vi "set_temperature_value.vi"   [LabVIEW 2019]
uses:
  global_temperature_cluster.ctl
  Instrument_Setup.vi
  Global/Global Variables/Data_Display_global.vi
  Global_temperature_variables.vi
types:
  T1 = typedef "global_temperature_cluster.ctl" = cluster{"370-T1":dbl, "370-T2":dbl, "370-T3":dbl, "370-T4":dbl, "370-T5":dbl, "372-T1":dbl, "372-T2":dbl, "372-T3":dbl, "372-T4":dbl, "372-T5":dbl, "372-T6":dbl, "350-T1":dbl, "350-T2":dbl, "350-T3":dbl, "350-T4":dbl, "VTI CH1":dbl, "VTI CH2":dbl, "VTI CH3":dbl, "AVS Control Channel (K)":dbl}
  T2 = typedef "PicowattAVS47-Cluster.ctl" = cluster{"Control Channel (K)":dbl, "AVS CH 5 (Res)":dbl, "AVS CH 6 (Res) ":dbl, "AVS CH 7 (Res) ":dbl, "Control Res.":dbl, "Auto Excitation":bool, "Auto activatet":bool, "AVS Excitation":i16}
  T3 = typedef "ITC503Monitor-Cluster.ctl" = cluster{"Temperatur (K)":dbl, "Setpoint (K)":dbl, "Rate (K/min)":dbl, "Heater (%)":dbl, "NV (%)":dbl, "Heater Manual":bool, "NV Manual":bool, "Go to Set":bool, "Heater SP":dbl, "Valid?":bool, "Set Heater SP":bool, "Set NV SP":bool, "Heater (%) Display":dbl, "NV (%) Display":dbl, "NV Setpoint":dbl, "Change Heater Status":bool, "Change NV Status":bool, "Sample 3":dbl, "Sample 2":dbl, "Sweep-State":bool, "Set Auto PID":bool, "Auto PID":bool, "Stopp":bool, "Setpoint-Sweep":dbl, "Sample 1":dbl, "Control Channel":bool, "Channel 1":bool, "Channel 2":bool, "Channel 3":bool}
  T4 = typedef "LS370_only_readout_cluster.ctl" = cluster{"LS370 T1":dbl, "LS370 T2":dbl, "LS370 T3":dbl, "LS370 T4":dbl, "LS370 T5":dbl, "LS370 R1":dbl, "LS370 R2":dbl, "LS370 R3":dbl, "LS370 R4":dbl, "LS370 R5":dbl, "LS370 T6":dbl, "LS370 T7":dbl, "LS370 T8":dbl, "LS370 T9":dbl, "LS370 R6":dbl, "LS370 R7":dbl, "LS370 R8":dbl, "LS370 R9":dbl, "LS370 TC-T":dbl, "LS370 TC-R":dbl, "Update Lakeshores":bool}
  T5 = typedef "LS372_read_only-Cluster.ctl" = cluster{"LS372-T1":dbl, "LS372 -T2":dbl, "LS372-T4":dbl, "LS372-T5":dbl, "LS372-T6":dbl, "LS372-R1 ":dbl, "LS372-R2":dbl, "LS372-R3 ":dbl, "LS372-R4 \n\n\n\n":dbl, "LS372-R5":dbl, "LS372-R6 ":dbl, "LS372-T3":dbl, "Update Lakeshores":bool}
  T6 = typedef "LS350-cluster.ctl" = cluster{"Setpoint":dbl, "Heater Output":dbl, "Setpoint control":dbl, "Enable Setpoint":bool, "LS350 T1":dbl, "LS350 T2":dbl, "LS350 T3":dbl, "LS350 T4":dbl, "LS350 R1":dbl, "LS350 R2":dbl, "LS350 R3":dbl, "LS350 R4":dbl}
  T7 = typedef "VTI-cluster.ctl" = cluster{"Temperatur (K)":dbl, "Setpoint (K)":dbl, "Rate (K/min)":dbl, "Heater (%)":dbl, "NV (%)":dbl, "Heater Manual":bool, "NV Manual":bool, "Go to Set":bool, "Pressure":dbl, "Heater SP":dbl, "Valid?":bool, "Set Heater SP":bool, "Set NV SP":bool, "Heater (%) Display":dbl, "NV (%) Display":dbl, "NV Setpoint":dbl, "Change Heater Status":bool, "Change NV Status":bool, "Sample 3":dbl, "Sample 2":dbl, "Sweep-State":bool, "Set Auto PID":bool, "Auto PID":bool, "Stopp":bool, "Setpoint-Sweep":dbl}
  T8 = typedef "LS370_Status.ctl" = cluster{"Setpoint":dbl, "MC Heater Output":dbl, "Still Heater Output":dbl, "Sorb  Heater Output":dbl, "LS370 T1":dbl, "LS370 T2":dbl, "LS370 T3":dbl, "LS370 T4":dbl, "LS370 T5":dbl, "LS370 R1":dbl, "LS370 R2":dbl, "LS370 R3":dbl, "LS370 R4":dbl, "LS370 R5":dbl, "LS370 T6":dbl, "LS370 T7":dbl, "LS370 T8":dbl, "LS370 T9":dbl, "LS370 R6":dbl, "LS370 R7":dbl, "LS370 R8":dbl, "LS370 R9":dbl, "LS370 TC-T":dbl, "LS370 TC-R":dbl}
  T9 = typedef "LS372-Cluster.ctl" = cluster{"Activate Tsweep":bool, "Setpoint - Manual":dbl, "Rate (K/min)":dbl, "Update Lakeshores":bool, "Still Heater":bool, "Still Power (mW)":dbl, "Manual Heater":bool, "Manual Heater  (mW) ":dbl, "Heater Range":dbl, "P (Gain)":dbl, "I (Reset)":dbl, "D (Rate)":dbl, "Heater Power (mW)":dbl, "MC Thermometer":u16, "MC Temperature":dbl, "LS372-T1":dbl, "LS372 -T2":dbl, "LS372-R1 ":dbl, "LS372-R2":dbl, "LS372-T3":dbl, "LS372-T4":dbl, "LS372-R3 ":dbl, "LS372-R4 \n\n\n\n":dbl, "LS372-T5":dbl, "LS372-T6":dbl, "LS372-R5":dbl, "LS372-R6 ":dbl, "Still Power ist":dbl, "Set Temperatur Sweep main":bool, "Setpoint ist":dbl, "Disable Heater":bool}
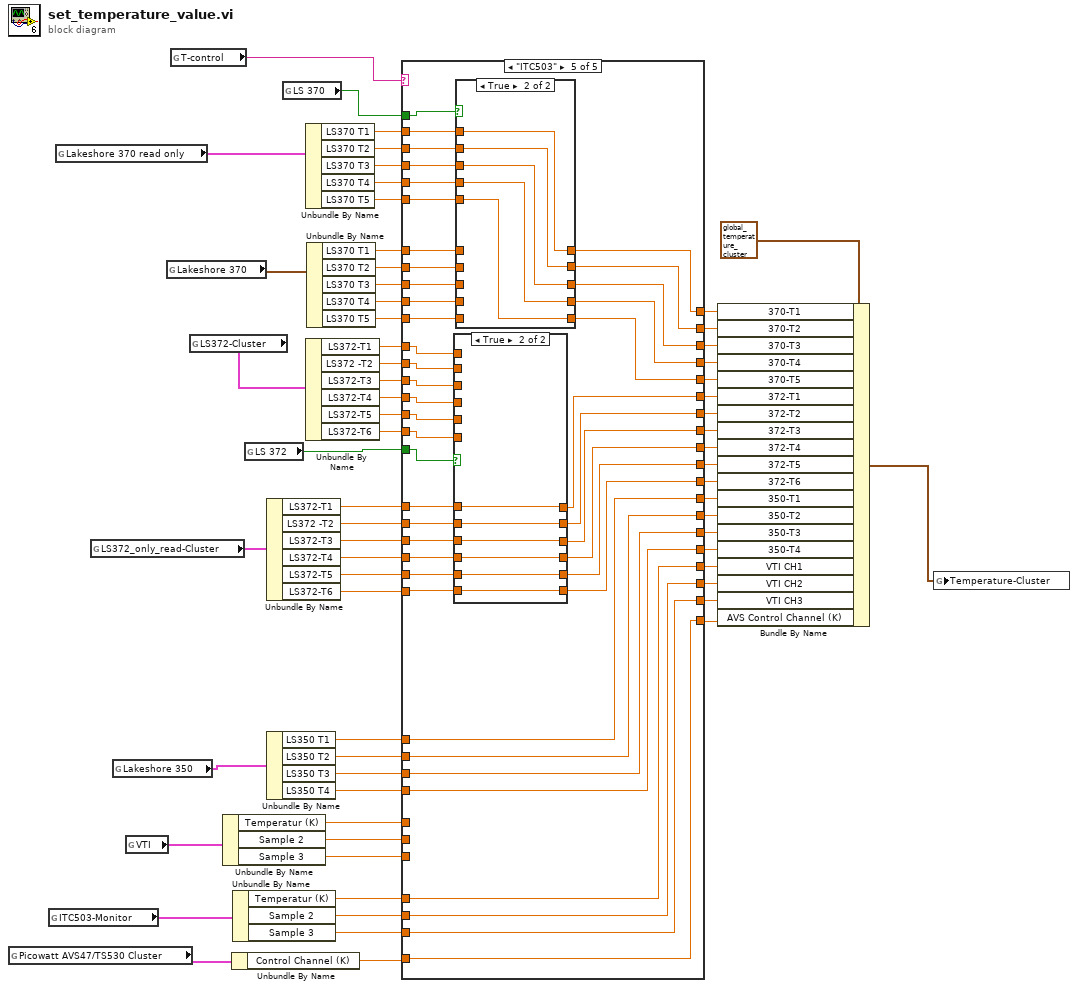
[diagram p0: block diagram]
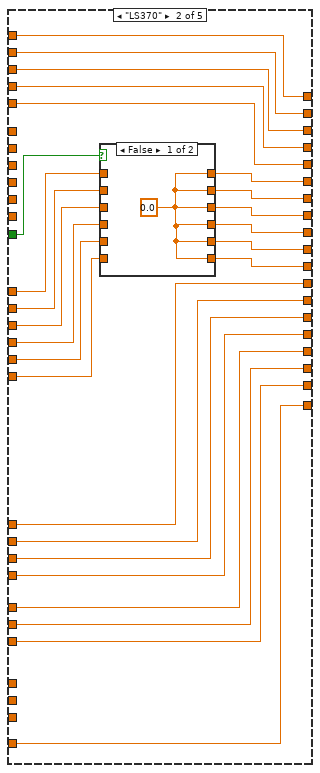
[diagram p5: hidden frame]
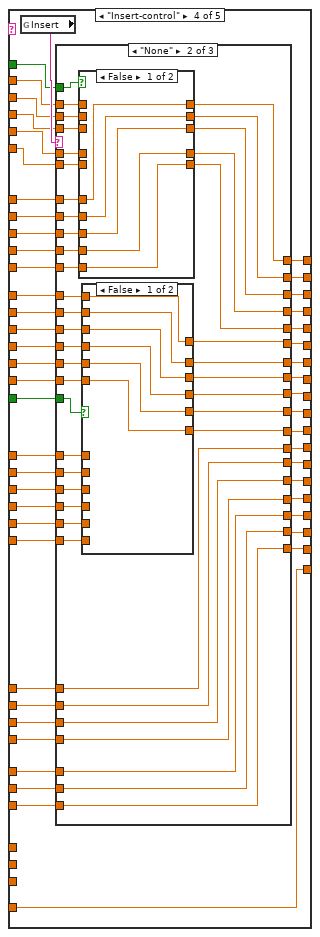
[diagram p9: hidden frame]
diagram:
  n1 = global read "Data_Display_global.vi" "Picowatt AVS47/TS530 Cluster"() -> (w56:T2)
  n2 = global read "Data_Display_global.vi" "ITC503-Monitor"() -> (w32:T3)
  n3 = global read "Data_Display_global.vi" "Lakeshore 370 read only"() -> (w7:T4)
  n4 = global read "Data_Display_global.vi" "LS372_only_read-Cluster"() -> (w57:T5)
  n5 = global read "Data_Display_global.vi" "Lakeshore 350"() -> (w58:T6)
  n6 = global read "Data_Display_global.vi" "VTI"() -> (w59:T7)
  n7 = global read "Data_Display_global.vi" "Lakeshore 370"() -> (w60:T8)
  n8 = global read "Instrument_Setup.vi" "T-control"() -> (w63:string)
  n9 = global read "Data_Display_global.vi" "LS372-Cluster"() -> (w61:T9)
  n10 = Unbundle By Name(w59) -> ("Temperatur (K)"=w33:dbl, "Sample 2"=w34:dbl, "Sample 3"=w35:dbl)
  n11 = Unbundle By Name(w56) -> ("Control Channel (K)"=w36:dbl)
  n12 = Unbundle By Name(w32) -> ("Temperatur (K)"=w31:dbl, "Sample 2"=w30:dbl, "Sample 3"=w29:dbl)
  n13 = global read "Instrument_Setup.vi" "LS 372"() -> (w62:bool)
  n14 = Unbundle By Name(w57) -> ("LS372-T1"=w17:dbl, "LS372 -T2"=w16:dbl, "LS372-T3"=w15:dbl, "LS372-T4"=w14:dbl, "LS372-T5"=w13:dbl, "LS372-T6"=w12:dbl)
  n15 = Unbundle By Name(w58) -> ("LS350 T1"=w11:dbl, "LS350 T2"=w10:dbl, "LS350 T3"=w9:dbl, "LS350 T4"=w8:dbl)
  n16 = global read "Instrument_Setup.vi" "LS 370"() -> (w1:bool)
  n17 = Unbundle By Name(w7) -> ("LS370 T1"=w6:dbl, "LS370 T2"=w5:dbl, "LS370 T3"=w4:dbl, "LS370 T4"=w3:dbl, "LS370 T5"=w2:dbl)
  n18 = Unbundle By Name(w61) -> ("LS372-T1"=w23:dbl, "LS372 -T2"=w22:dbl, "LS372-T3"=w21:dbl, "LS372-T4"=w20:dbl, "LS372-T5"=w19:dbl, "LS372-T6"=w18:dbl)
  n19 = Unbundle By Name(w60) -> ("LS370 T1"=w28:dbl, "LS370 T2"=w27:dbl, "LS370 T3"=w26:dbl, "LS370 T4"=w25:dbl, "LS370 T5"=w24:dbl)
  n20 = case shown="\"ITC503\"" w63 {
    tunnel: w62 -> [w92 w156 _ w248 w452]
    tunnel: [w97 w151 w187 w235 w457] -> w55
    tunnel: [w96 w150 w186 w234 w456] -> w54
    tunnel: [w95 w149 w185 w233 w455] -> w53
    tunnel: [w94 w148 w184 w232 w454] -> w52
    tunnel: [w93 w147 w183 w231 w453] -> w51
    tunnel: [w79 w146 w177 w230 w439] -> w50
    tunnel: [w78 w145 w176 w229 w438] -> w49
    tunnel: [w77 w144 w175 w228 w437] -> w48
    tunnel: [w76 w143 w174 w227 w436] -> w47
    tunnel: [w75 w142 w173 w226 w435] -> w46
    tunnel: [w74 w141 w172 w225 w434] -> w45
    tunnel: [w73 w140 w171 w217 w433] -> w44
    tunnel: [w72 w137 w170 w216 w432] -> w43
    tunnel: [w71 w139 w169 w215 w431] -> w42
    tunnel: [w70 w138 w168 w214 w430] -> w41
    tunnel: [w69 w152 w167 w213 w429] -> w40
    tunnel: [w68 w153 w166 w212 w428] -> w39
    tunnel: [w67 w154 w165 w211 w427] -> w38
    tunnel: [w66 w155 w164 w210 w426] -> w37
    tunnel: w36 -> [w66 w155 w164 w210 w426]
    tunnel: w35 -> [w67 w154 w165 w218 _]
    tunnel: w34 -> [w68 w153 w166 w219 _]
    tunnel: w33 -> [w69 w152 w167 w220 _]
    tunnel: w31 -> [_ _ _ _ w429]
    tunnel: w30 -> [_ _ _ _ w428]
    tunnel: w29 -> [_ _ _ _ w427]
    tunnel: w28 -> [w102 w151 w182 w253 w462]
    tunnel: w27 -> [w101 w150 w181 w252 w461]
    tunnel: w26 -> [w100 w149 w180 w251 w460]
    tunnel: w25 -> [w99 w148 w179 w250 w459]
    tunnel: w24 -> [w98 w147 w178 w249 w458]
    tunnel: w23 -> [w91 _ w177 w247 w451]
    tunnel: w22 -> [w90 _ w176 w246 w450]
    tunnel: w21 -> [w89 _ w175 w245 w449]
    tunnel: w20 -> [w88 _ w174 w244 w448]
    tunnel: w19 -> [w87 _ w173 w243 w447]
    tunnel: w18 -> [w86 _ w172 w242 w446]
    tunnel: w17 -> [w85 w131 _ w241 w445]
    tunnel: w16 -> [w84 w132 _ w240 w444]
    tunnel: w15 -> [w83 w133 _ w239 w443]
    tunnel: w14 -> [w82 w134 _ w238 w442]
    tunnel: w13 -> [w81 w135 _ w237 w441]
    tunnel: w12 -> [w80 w136 _ w236 w440]
    tunnel: w11 -> [w73 w140 w171 w224 w433]
    tunnel: w10 -> [w72 w137 w170 w223 w432]
    tunnel: w9 -> [w71 w139 w169 w222 w431]
    tunnel: w8 -> [w70 w138 w168 w221 w430]
    tunnel: w6 -> [w107 _ w192 w208 w467]
    tunnel: w5 -> [w106 _ w191 w207 w466]
    tunnel: w4 -> [w105 _ w190 w206 w465]
    tunnel: w3 -> [w104 _ w189 w205 w464]
    tunnel: w2 -> [w103 _ w188 w204 w463]
    tunnel: w1 -> [w108 _ w193 w209 w468]
    frame "None", Default {
      n21 = case shown="False" w92 {
        tunnel: w91 -> [w114 _]
        tunnel: w90 -> [w113 _]
        tunnel: w89 -> [w112 _]
        tunnel: w88 -> [w111 _]
        tunnel: w87 -> [w110 _]
        tunnel: w86 -> [w109 _]
        tunnel: w85 -> [_ w120]
        tunnel: w84 -> [_ w119]
        tunnel: w83 -> [_ w118]
        tunnel: w82 -> [_ w117]
        tunnel: w81 -> [_ w116]
        tunnel: w80 -> [_ w115]
        tunnel: [w114 w120] -> w79
        tunnel: [w113 w119] -> w78
        tunnel: [w112 w118] -> w77
        tunnel: [w111 w117] -> w76
        tunnel: [w110 w116] -> w75
        tunnel: [w109 w115] -> w74
        frame False {
        }
        frame True {
        }
      }
      n22 = case shown="False" w108 {
        tunnel: w107 -> [_ w130]
        tunnel: w106 -> [_ w129]
        tunnel: w105 -> [_ w128]
        tunnel: w104 -> [_ w127]
        tunnel: w103 -> [_ w126]
        tunnel: [w125 w130] -> w97
        tunnel: [w124 w129] -> w96
        tunnel: [w123 w128] -> w95
        tunnel: [w122 w127] -> w94
        tunnel: [w121 w126] -> w93
        tunnel: w102 -> [w125 _]
        tunnel: w101 -> [w124 _]
        tunnel: w100 -> [w123 _]
        tunnel: w99 -> [w122 _]
        tunnel: w98 -> [w121 _]
        frame False {
        }
        frame True {
        }
      }
    }
    frame "LS370" {
      n23 = case shown="False" w156 {
        tunnel: w131 -> [_ w163]
        tunnel: w132 -> [_ w162]
        tunnel: w133 -> [_ w161]
        tunnel: w134 -> [_ w160]
        tunnel: w135 -> [_ w159]
        tunnel: w136 -> [_ w158]
        tunnel: [w157 w163] -> w146
        tunnel: [w157 w162] -> w145
        tunnel: [w157 w161] -> w144
        tunnel: [w157 w160] -> w143
        tunnel: [w157 w159] -> w142
        tunnel: [w157 w158] -> w141
        frame False {
          w157 = 0.0
        }
        frame True {
        }
      }
    }
    frame "LS372" {
      n24 = case shown="False" w193 {
        tunnel: w192 -> [_ w203]
        tunnel: w191 -> [_ w202]
        tunnel: w190 -> [_ w201]
        tunnel: w189 -> [_ w200]
        tunnel: w188 -> [_ w199]
        tunnel: [w198 w203] -> w187
        tunnel: [w197 w202] -> w186
        tunnel: [w196 w201] -> w185
        tunnel: [w195 w200] -> w184
        tunnel: [w194 w199] -> w183
        tunnel: w182 -> [w198 _]
        tunnel: w181 -> [w197 _]
        tunnel: w180 -> [w196 _]
        tunnel: w179 -> [w195 _]
        tunnel: w178 -> [w194 _]
        frame False {
        }
        frame True {
        }
      }
    }
    frame "Insert-control" {
      n25 = global read "Instrument_Setup.vi" "Insert"() -> (w254:string)
      n26 = case shown="\"None\"" w254 {
        tunnel: w253 -> [w290 w354 w400]
        tunnel: w252 -> [w289 w353 w399]
        tunnel: w251 -> [w288 w352 w398]
        tunnel: w250 -> [w287 w351 w397]
        tunnel: w249 -> [w286 w350 w396]
        tunnel: w248 -> [w274 w344 w413]
        tunnel: w247 -> [w280 w343 w412]
        tunnel: w246 -> [w279 w342 w411]
        tunnel: w245 -> [w278 w341 w410]
        tunnel: w244 -> [w277 w340 w409]
        tunnel: w243 -> [w276 w339 w408]
        tunnel: w242 -> [w275 w338 w407]
        tunnel: w241 -> [w273 w337 w406]
        tunnel: w240 -> [w272 w336 w405]
        tunnel: w239 -> [w271 w335 w404]
        tunnel: w238 -> [w270 w334 w403]
        tunnel: w237 -> [w269 w333 w402]
        tunnel: w236 -> [w268 w332 w401]
        tunnel: [w285 w349 w400] -> w235
        tunnel: [w284 w348 w399] -> w234
        tunnel: [w283 w347 w398] -> w233
        tunnel: [w282 w346 w397] -> w232
        tunnel: [w281 w345 w396] -> w231
        tunnel: [w267 w331 w395] -> w230
        tunnel: [w266 w330 w394] -> w229
        tunnel: [w265 w329 w393] -> w228
        tunnel: [w264 w328 w392] -> w227
        tunnel: [w263 w327 w391] -> w226
        tunnel: [w262 w326 w390] -> w225
        tunnel: w224 -> [w261 w325 w389]
        tunnel: w223 -> [w260 w324 w388]
        tunnel: w222 -> [w259 w323 w387]
        tunnel: w221 -> [w258 w322 w386]
        tunnel: [w261 w325 w389] -> w217
        tunnel: [w260 w324 w388] -> w216
        tunnel: [w259 w323 w387] -> w215
        tunnel: [w258 w322 w386] -> w214
        tunnel: w220 -> [w257 w321 w385]
        tunnel: w219 -> [w256 w320 w384]
        tunnel: w218 -> [w255 w319 w383]
        tunnel: [w257 w321 w385] -> w213
        tunnel: [w256 w320 w384] -> w212
        tunnel: [w255 w319 w383] -> w211
        tunnel: w209 -> [w296 w360 _]
        tunnel: w208 -> [w295 w359 _]
        tunnel: w207 -> [w294 w358 _]
        tunnel: w206 -> [w293 w357 _]
        tunnel: w205 -> [w292 w356 _]
        tunnel: w204 -> [w291 w355 _]
        frame "VTI", Default {
          n27 = case shown="False" w296 {
            tunnel: w295 -> [_ w318]
            tunnel: w294 -> [_ w317]
            tunnel: w293 -> [_ w316]
            tunnel: w292 -> [_ w315]
            tunnel: w291 -> [_ w314]
            tunnel: w290 -> [w313 _]
            tunnel: w289 -> [w312 _]
            tunnel: w288 -> [w311 _]
            tunnel: w287 -> [w310 _]
            tunnel: w286 -> [w309 _]
            tunnel: [w313 w318] -> w285
            tunnel: [w312 w317] -> w284
            tunnel: [w311 w316] -> w283
            tunnel: [w310 w315] -> w282
            tunnel: [w309 w314] -> w281
            frame False {
            }
            frame True {
            }
          }
          n28 = case shown="True" w274 {
            tunnel: w280 -> [w302 _]
            tunnel: w279 -> [w301 _]
            tunnel: w278 -> [w300 _]
            tunnel: w277 -> [w299 _]
            tunnel: w276 -> [w298 _]
            tunnel: w275 -> [w297 _]
            tunnel: w273 -> [_ w308]
            tunnel: w272 -> [_ w307]
            tunnel: w271 -> [_ w306]
            tunnel: w270 -> [_ w305]
            tunnel: w269 -> [_ w304]
            tunnel: w268 -> [_ w303]
            tunnel: [w302 w308] -> w267
            tunnel: [w301 w307] -> w266
            tunnel: [w300 w306] -> w265
            tunnel: [w299 w305] -> w264
            tunnel: [w298 w304] -> w263
            tunnel: [w297 w303] -> w262
            frame False {
            }
            frame True {
            }
          }
        }
        frame "None" {
          n29 = case shown="False" w360 {
            tunnel: w359 -> [_ w382]
            tunnel: w358 -> [_ w381]
            tunnel: w357 -> [_ w380]
            tunnel: w356 -> [_ w379]
            tunnel: w355 -> [_ w378]
            tunnel: w354 -> [w377 _]
            tunnel: w353 -> [w376 _]
            tunnel: w352 -> [w375 _]
            tunnel: w351 -> [w374 _]
            tunnel: w350 -> [w373 _]
            tunnel: [w377 w382] -> w349
            tunnel: [w376 w381] -> w348
            tunnel: [w375 w380] -> w347
            tunnel: [w374 w379] -> w346
            tunnel: [w373 w378] -> w345
            frame False {
            }
            frame True {
            }
          }
          n30 = case shown="False" w344 {
            tunnel: w343 -> [w366 _]
            tunnel: w342 -> [w365 _]
            tunnel: w341 -> [w364 _]
            tunnel: w340 -> [w363 _]
            tunnel: w339 -> [w362 _]
            tunnel: w338 -> [w361 _]
            tunnel: w337 -> [_ w372]
            tunnel: w336 -> [_ w371]
            tunnel: w335 -> [_ w370]
            tunnel: w334 -> [_ w369]
            tunnel: w333 -> [_ w368]
            tunnel: w332 -> [_ w367]
            tunnel: [w366 w372] -> w331
            tunnel: [w365 w371] -> w330
            tunnel: [w364 w370] -> w329
            tunnel: [w363 w369] -> w328
            tunnel: [w362 w368] -> w327
            tunnel: [w361 w367] -> w326
            frame False {
            }
            frame True {
            }
          }
        }
        frame "JT" {
          n31 = case shown="False" w413 {
            tunnel: w412 -> [w419 _]
            tunnel: w411 -> [w418 _]
            tunnel: w410 -> [w417 _]
            tunnel: w409 -> [w416 _]
            tunnel: w408 -> [w415 _]
            tunnel: w407 -> [w414 _]
            tunnel: w406 -> [_ w425]
            tunnel: w405 -> [_ w424]
            tunnel: w404 -> [_ w423]
            tunnel: w403 -> [_ w422]
            tunnel: w402 -> [_ w421]
            tunnel: w401 -> [_ w420]
            tunnel: [w419 w425] -> w395
            tunnel: [w418 w424] -> w394
            tunnel: [w417 w423] -> w393
            tunnel: [w416 w422] -> w392
            tunnel: [w415 w421] -> w391
            tunnel: [w414 w420] -> w390
            frame False {
            }
            frame True {
            }
          }
        }
      }
    }
    frame "ITC503" {
      n32 = case shown="True" w452 {
        tunnel: w451 -> [w474 _]
        tunnel: w450 -> [w473 _]
        tunnel: w449 -> [w472 _]
        tunnel: w448 -> [w471 _]
        tunnel: w447 -> [w470 _]
        tunnel: w446 -> [w469 _]
        tunnel: w445 -> [_ w480]
        tunnel: w444 -> [_ w479]
        tunnel: w443 -> [_ w478]
        tunnel: w442 -> [_ w477]
        tunnel: w441 -> [_ w476]
        tunnel: w440 -> [_ w475]
        tunnel: [w474 w480] -> w439
        tunnel: [w473 w479] -> w438
        tunnel: [w472 w478] -> w437
        tunnel: [w471 w477] -> w436
        tunnel: [w470 w476] -> w435
        tunnel: [w469 w475] -> w434
        frame False {
        }
        frame True {
        }
      }
      n33 = case shown="True" w468 {
        tunnel: w467 -> [_ w490]
        tunnel: w466 -> [_ w489]
        tunnel: w465 -> [_ w488]
        tunnel: w464 -> [_ w487]
        tunnel: w463 -> [_ w486]
        tunnel: w462 -> [w485 _]
        tunnel: w461 -> [w484 _]
        tunnel: w460 -> [w483 _]
        tunnel: w459 -> [w482 _]
        tunnel: w458 -> [w481 _]
        tunnel: [w485 w490] -> w457
        tunnel: [w484 w489] -> w456
        tunnel: [w483 w488] -> w455
        tunnel: [w482 w487] -> w454
        tunnel: [w481 w486] -> w453
        frame False {
        }
        frame True {
        }
      }
    }
  }
  n34 = Bundle By Name(cluster=T1 {"370-T1"=0.0, "370-T2"=0.0, "370-T3"=0.0, "370-T4"=0.0, "370-T5"=0.0, "372-T1"=0.0, "372-T2"=0.0, "372-T3"=0.0, "372-T4"=0.0, "372-T5"=0.0, "372-T6"=0.0, "350-T1"=0.0, "350-T2"=0.0, "350-T3"=0.0, "350-T4"=0.0, "VTI CH1"=0.0, "VTI CH2"=0.0, "VTI CH3"=0.0, "AVS Control Channel (K)"=0.0} ("Temperature-Cluster"), "370-T1"=w55, "370-T2"=w54, "370-T3"=w53, "370-T4"=w52, "370-T5"=w51, "372-T1"=w50, "372-T2"=w49, "372-T3"=w48, "372-T4"=w47, "372-T5"=w46, "372-T6"=w45, "350-T1"=w44, "350-T2"=w43, "350-T3"=w42, "350-T4"=w41, "VTI CH1"=w40, "VTI CH2"=w39, "VTI CH3"=w38, "AVS Control Channel (K)"=w37) -> (w64:T1)
  n35 = global write "Global_temperature_variables.vi" "Temperature-Cluster"(w64) -> ()
